vi "Method.vi"(8 "error in (no error)":errorcluster, 11 "First Library in":refnum<class "First Library.lvclass">) -> (0 "error out":errorcluster, 3 "First Library out":refnum<class "First Library.lvclass">)   [LabVIEW 2021, in "_Create From Template.lvlib" / "Templates.lvlib" / "First Library.lvlib" / "First Library.lvclass"]
uses:
  First Library.lvclass
  First Library.lvclass/First Library.ctl
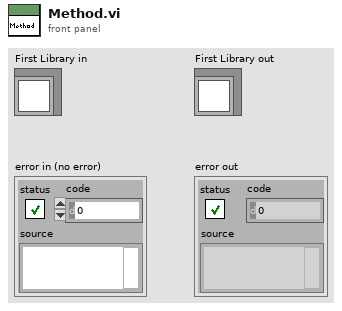
[diagram p1: front panel]
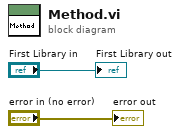
[diagram p0: block diagram]
diagram:
  "error out" <- "error in (no error)"
  "First Library out" <- "First Library in"
